vi "Next JSON Value.vi"(10 "Offset":i32, 11 "JSON":string) -> (1 "<JSON>":string caption="<JSON>Value", 2 "Offset past":i32 caption="Offset past Value", 3 "Rest of Input String":string, 4 "JSON Value Type":T1)   [LabVIEW 2019, in "JSONtext.lvlib"]
doc: "Gets the next JSON Value (object, array, string, number, true, false, or null)\n\n\"Offset\" should point to the start of the JSON Value, or to whitespace in front of the Value."
uses:
  JSONtext.lvlib
  JSON Value Type.ctl
  Parsing/Parsing State.ctl
  Parsing/Advance past whitespace.vi
  Parsing/Advance past String.vi
  Parsing/Advance past Number.vi
  Parsing/Advance past Line Ending.vi
  Parsing/Advance past Array.vi
  Parsing/Advance past Object.vi
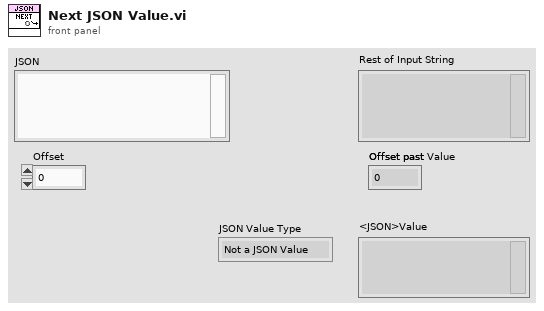
[diagram p1: front panel]
types:
  T1 = typedef "JSONtext.lvlib/JSON Value Type.ctl" = enum16{"Not a JSON Value", "JSON Object", "JSON Array", "String", "Number", "true", "false", "null"}
  T2 = typedef "JSONtext.lvlib/Parsing State.ctl" = enum16{"Parser Error", "Object", "Array", "String", "Number/Other", "Leading Whitespace", "Object end", "Array end", "Value end"}
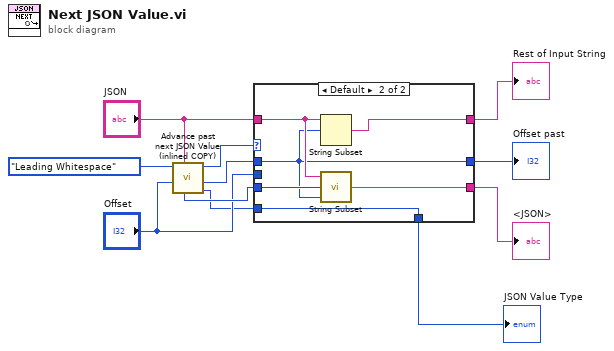
[diagram p0: block diagram]
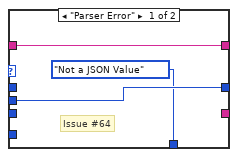
[diagram p2: hidden frame]
diagram:
  n1 = call "Advance past next JSON Value (inlined COPY).vi"("JSON"="JSON", "Offset"="Offset", "State"=Parsing_State."Leading Whitespace" ("Parser State in")) -> ("JSON Value Type"=w1:T1, "Offset"=w8:i32, "State"=w4:T2, "Value start"=w10:i32)  [unwired: 4 in, 1 out]
  n2 = case shown="Default" w4 {
    tunnel: w10 -> [_ w20]
    tunnel: "Offset" -> [w13 _]
    tunnel: w8 -> [_ w16]
    tunnel: [_ w19] -> w7
    tunnel: "JSON" -> [w14 w18]
    tunnel: [w14 w17] -> w5
    tunnel: [w13 w16] -> w3
    tunnel: [JSON_Value_Type."Not a JSON Value" ("JSON Value Type") w15] -> w2
    tunnel: w1 -> [_ w15]
    frame "Parser Error" {
      # "Issue #64"
    }
    frame Default {
      n3 = String Subset(string=w18, offset (0)=w16) -> (substring=w17:string)  [unwired: 1 in]
      n4 = call "String Subset.vi"("Offset past End"=w16, "Start offset"=w20, "JSON"=w18) -> ("substring"=w19:string)  [unwired: 2 in]
    }
  }
  "JSON Value Type" <- w2
  "Rest of Input String" <- w5
  "<JSON>" <- w7
  "Offset past" <- w3
